vi "Write Multiple Holding Registers.vi"(8 "error in (no error)":errorcluster caption="错误输入（无错误）", 9 "holding register values":u16[](array[numeric]) caption="保持寄存器值", 10 "starting address":u16 caption="起始地址", 11 "Modbus master in":refnum<class "Modbus Master.lvclass"> caption="Modbus主设备输入") -> (0 "error out":errorcluster caption="错误输出", 3 "Modbus master out":refnum<class "Modbus Master.lvclass"> caption="Modbus主设备输出")   [LabVIEW 2014, in "Modbus Master.lvclass"]
doc: "写入值至连续保持寄存器。VI可写入的最大保持寄存器数量为123。"
uses:
  <vilib>/Modbus/master/Modbus Master.lvclass
  <vilib>/Modbus/subvis/Modbus API/Modbus API.lvclass/Modbus API.ctl
  <vilib>/Modbus/master/Modbus Master.lvclass/Modbus Master.ctl
  <vilib>/Modbus/subvis/Protocol/Interfaces/Network Master/Network Master.lvclass
  <vilib>/Modbus/subvis/Transmission Data Unit (ADU)/Transmission Data Unit/Transmission Data Unit.lvclass
  <vilib>/Modbus/subvis/Data and Functions/Master Function Definition/Master Function Definition.lvlib
  <vilib>/Modbus/subvis/Modbus API/Modbus API.lvclass
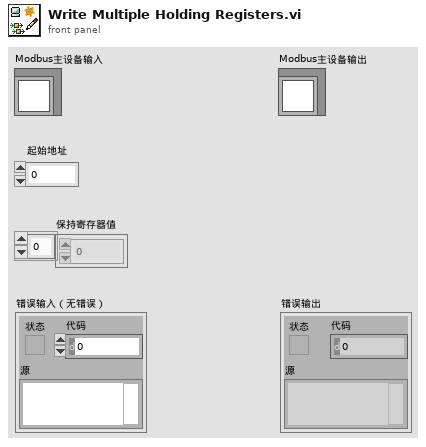
[diagram p1: front panel]
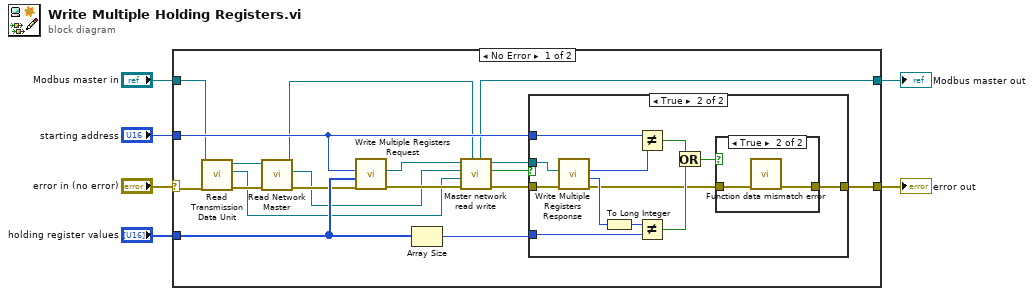
[diagram p0: block diagram]
diagram:
  n1 = case shown="No Error" "error in (no error)" {
    selector: "error in (no error)" -> [w7 w42]
    tunnel: "Modbus master in" -> [w8 w41]
    tunnel: [w23 w42] -> w3
    tunnel: [w16 w41] -> w4
    tunnel: "holding register values" -> [w20 _]
    tunnel: "starting address" -> [w22 _]
    frame No Error {
      n2 = call <vilib>:"Read Transmission Data Unit.vi"("error in (no error)"=w7, "Modbus instance in"=w8) -> ("error out"=w15:errorcluster, "transmission data unit"=w10:refnum<class "Transmission Data Unit.lvclass">, "Modbus instance out"=w13:refnum<class "Modbus Master.lvclass">)  [unwired: 7 in]
      n3 = call <vilib>:"Read Network Master.vi"("error in (no error)"=w15, "Modbus master in"=w13) -> ("error out"=w14:errorcluster, "network master"=w11:refnum<class "Network Master.lvclass">, "Modbus master out"=w12:refnum<class "Modbus Master.lvclass">)  [unwired: 7 in]
      n4 = call <vilib>:"Write Multiple Registers Request.vi"("error in (no error)"=w14, "registers"=w20, "starting address"=w22) -> ("error out"=w24:errorcluster, "Modbus data unit out"=w18:refnum<class "Modbus Data Unit (PDU).lvclass">)  [unwired: 7 in]
      n5 = Array Size(array=w20) -> (size(s)=w21:i32)
      n6 = call <vilib>:"Master network read write.vi"("Modbus master in"=w12, "error in (no error)"=w24, "transmission data unit in"=w10, "network master in"=w11, "Modbus data unit in"=w18) -> ("error out"=w19:errorcluster, "PDU valid?"=w9:bool, "Modbus data unit out"=w17:refnum<class "Modbus Data Unit (PDU).lvclass">, "Modbus master out"=w16:refnum<class "Modbus Master.lvclass">)  [unwired: 3 in]
      n7 = case shown="True" w9 {
        tunnel: [w25 w34] -> w23
        tunnel: w22 -> [_ w27]
        tunnel: w21 -> [_ w32]
        tunnel: w19 -> [w25 w31]
        tunnel: w17 -> [_ w30]
        frame False {
        }
        frame True {
          n8 = call <vilib>:"Write Multiple Registers Response.vi"("error in (no error)"=w31, "Modbus data unit in"=w30) -> ("error out"=w29:errorcluster, "number of registers"=w33:u16, "start address"=w28:u16)  [unwired: 7 in]
          n9 = To Long Integer(number=w33) -> (32bit integer=w26:i32)
          n10 = Not Equal?(x=w27, y=w28) -> (x != y?=w36:bool)
          n11 = Not Equal?(x=w26, y=w32) -> (x != y?=w35:bool)
          n12 = Or(x=w36, y=w35) -> (x .or. y?=w37:bool)
          n13 = case shown="True" w37 {
            tunnel: [w38 w40] -> w34
            tunnel: w29 -> [w38 w39]
            frame False {
            }
            frame True {
              n14 = call <vilib>:"Function data mismatch error.vi"("error in (no error)"=w39) -> ("error out"=w40:errorcluster)  [unwired: 10 in]
            }
          }
        }
      }
    }
    frame Error {
    }
  }
  "error out" <- w3
  "Modbus master out" <- w4
